vi "Build.vi"(4 "Build Specification Version":T1, 6 "Destination":path=path "Module Plugin Distribution", 7 "String in":refnum<vi>, 8 "error in":errorcluster, 9 "BuildSpecification":path=path "Module Plugin Distribution", 10 "Project":path=path "C:/temp/Workspace/Components/Modules/Data Collector Report Models/External/JSON/DC - JSON.lvproj", 11 "WorkspaceFolder":path=path "C:/temp/Workspace") -> (0 "error out":errorcluster)   [LabVIEW 2017]
uses:
  <vilib>/AppBuilder/AB_API_Simple/Build Specification Version.ctl
  <vilib>/AppBuilder/AB_API_Simple/Set Build Specification Version (path).vi
  <vilib>/AppBuilder/AB_API_Simple/Build (path).vi
  <vilib>/AppBuilder/AB_API/SDIST/NI_AB_API_SDIST.lvclass
  <vilib>/AppBuilder/AB_API/PPL/NI_AB_API_PPL.lvclass
  <vilib>/AppBuilder/AB_API_Simple/NI_App_Builder_API.lvlib
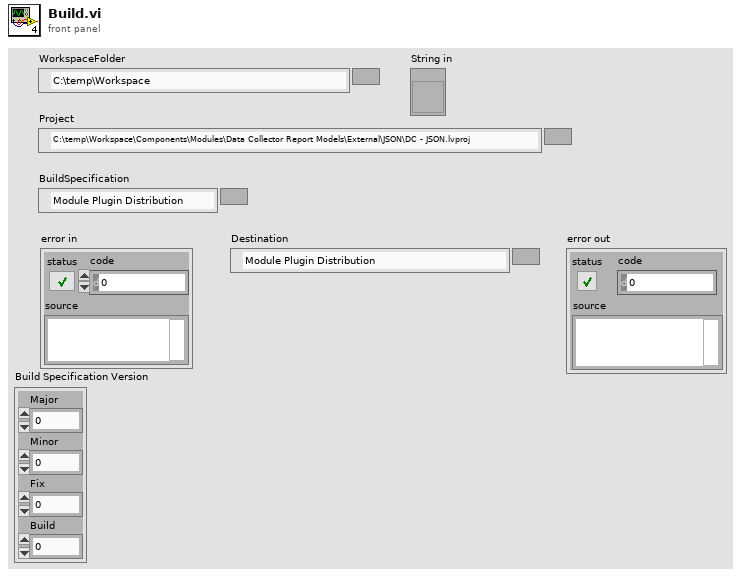
[diagram p1: front panel]
types:
  T1 = typedef "NI_App_Builder_API.lvlib/Build Specification Version.ctl" = cluster{"Major":u16, "Minor":u16, "Fix":u16, "Build":u16}
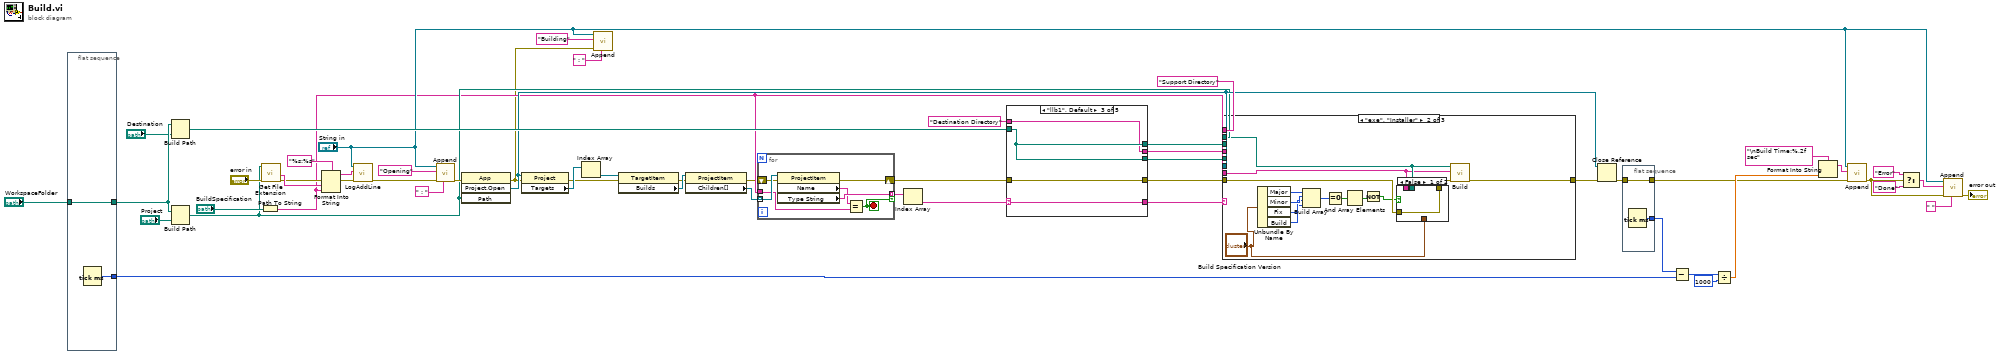
[diagram p0: block diagram]
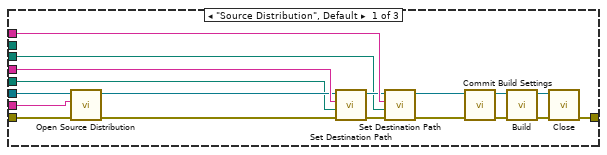
[diagram p2: hidden frame]
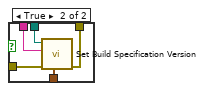
[diagram p3: hidden frame]
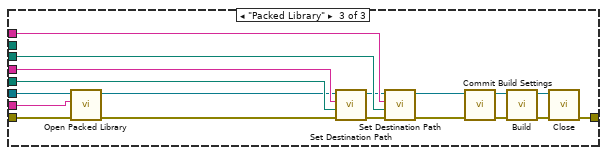
[diagram p4: hidden frame]
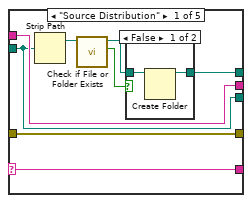
[diagram p5: hidden frame]
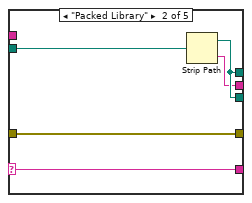
[diagram p7: hidden frame]
diagram:
  n1 = flat-sequence {
    tunnel: [w58] -> w25
    tunnel: "WorkspaceFolder" -> [w58]
    tunnel: [w57] -> w20
    frame #0 {
      n2 = Tick Count (ms)() -> (millisecond timer value=w57:u32)
    }
  }
  n3 = Build Path(base path=w25, name or relative path="Destination") -> (appended path=w47:path)
  n4 = Build Path(base path=w25, name or relative path="Project") -> (appended path=w12:path)
  n5 = Path To String(path="BuildSpecification") -> (string=w9:string)
  n6 = call <vilib>:"Get File Extension.vi"("error in (no error)"="error in", "file"=w12) -> ("error out"=w45:errorcluster, "filename without extension"=w50:string)  [unwired: 5 in, 3 out]
  n7 = Format Into String(format string="%s:%s", error in=w45, w50, w9) -> (resulting string=w28:string, error out=w30:errorcluster)  [unwired: 1 in]
  n8 = call "LogAddLine.vi"("error in (no error)"=w30, "Msg in"=w28, "String in"="String in") -> ("error out"=w29:errorcluster)  [unwired: 6 in, 1 out]
  n9 = call "Append.vi"("separator"=" : ", "error in (no error)"=w29, "Msg in"="Opening" ("format string"), "String in"="String in") -> ("error out"=w35:errorcluster)  [unwired: 6 in]
  n10 = invoke class="App" method="Project.Open"(error in=w35, "Path"=w12) -> (error out=w5:errorcluster, "Project:Open"=w39:refnum<vi>)  [unwired: 2 in, 2 out]
  n11 = property class="Project"(reference=w39, error in=w5) -> (error out=w4:errorcluster, "Targets"=w38:refnum<vi>[])  [unwired: 1 out]
  n12 = Index Array(array=w38) -> (element=w37:refnum<vi>)  [unwired: 1 in]
  n13 = call "Append.vi"("separator"=" : ", "error in (no error)"=w5, "Msg in"="Building" ("format string"), "String in"="String in") -> ()  [unwired: 6 in, 1 out]
  n14 = property class="TargetItem"(reference=w37, error in=w4) -> (error out=w3:errorcluster, "Builds"=w36:refnum<vi>)  [unwired: 1 out]
  n15 = property class="ProjectItem"(reference=w36, error in=w3) -> (error out=w2:errorcluster, "Children[]"=w10:refnum<vi>[])  [unwired: 1 out]
  n16 = for {
    tunnel: [w65] -> w8 mode=indexing if=w61
    tunnel: w10 -> [w64] mode=indexing
    tunnel: w9 -> [w62]
    shift-right: [w59] -> w1
    shift-left: w2 -> [w60]
    stop <- w61 stop-if-true
    n17 = property class="ProjectItem"(reference=w64, error in=w60) -> (error out=w59:errorcluster, "Name"=w63:string, "Type String"=w65:string)  [unwired: 1 out]
    n18 = Equal?(x=w63, y=w62) -> (x = y?=w61:bool)
  }
  n19 = Index Array(array=w8) -> (element=w7:string)  [unwired: 1 in]
  n20 = case shown="\"llb1\", Default" w7 {
    selector: w7 -> [w67 w78 w83 w87 w91]
    tunnel: [w72 w80 w85 w89 w92] -> w46
    tunnel: w47 -> [w72 w81 w85 w89 w92]
    tunnel: [w68 w80 w85 w89 w92] -> w44
    tunnel: [w67 w78 w83 w87 w91] -> w43
    tunnel: [w73 w79 w84 w88 w93] -> w41
    tunnel: "Destination Directory" ("Destination label") -> [w73 _ w84 w88 w93]
    tunnel: [w66 w77 w82 w86 w90] -> w6
    tunnel: w1 -> [w66 w77 w82 w86 w90]
    frame "Source Distribution" {
      n21 = Strip Path(path=w72) -> (stripped path=w69:path)  [unwired: 1 out]
      n22 = call <vilib>:"Check if File or Folder Exists.vi"("path"=w69) -> ("file or folder exists?"=w71:bool, "dup path"=w70:path)  [unwired: 8 in, 1 out]
      n23 = case shown="False" w71 {
        tunnel: w70 -> [w75 w76]
        tunnel: [w74 w76] -> w68
        frame False {
          n24 = Create Folder(path (use dialog)=w75) -> (created path=w74:path)  [unwired: 2 in, 2 out]
        }
        frame True {
        }
      }
    }
    frame "Packed Library" {
      n25 = Strip Path(path=w81) -> (stripped path=w80:path, name=w79:string)
    }
    frame "llb1", Default {
    }
    frame "exe" {
    }
    frame "" {
    }
  }
  n26 = case shown="\"exe\", \"Installer\"" w43 {
    tunnel: [w107 w125 w140] -> w42
    tunnel: w41 -> [w106 _ w148]
    tunnel: "Support Directory" ("Destination label") -> [w103 _ w146]
    tunnel: w46 -> [w98 _ w149]
    tunnel: w44 -> [w97 _ w145]
    tunnel: w6 -> [w96 w122 w139]
    tunnel: w39 -> [w95 _ w138]
    tunnel: w9 -> [w94 w123 w137]
    tunnel: w12 -> [_ w124 _]
    frame "Source Distribution", Default {
      n27 = call <vilib>:"Open Source Distribution.vi"("error in (no error)"=w96, "Build specification name"=w94, "Project Refnum"=w95) -> ("error out"=w104:errorcluster, "SDIST out"=w105:refnum<class "NI_AB_API_SDIST.lvclass">)  [unwired: 7 in]
      n28 = call-dynamic "Set Destination Path.vi"("error in (no error)"=w104, "Destination path"=w98, "Destination label"=w106, "SDIST in"=w105) -> ("error out"=w101:errorcluster, "SDIST out"=w102:refnum<class "NI_AB_API_SDIST.lvclass">)  [unwired: 6 in]
      n29 = call-dynamic "Set Destination Path.vi"("error in (no error)"=w101, "Destination path"=w97, "Destination label"=w103, "SDIST in"=w102) -> ("error out"=w100:errorcluster, "SDIST out"=w99:refnum<class "NI_AB_API_SDIST.lvclass">)  [unwired: 6 in]
      n30 = call-dynamic "Commit Build Settings.vi"("error in (no error)"=w100, "SDIST in"=w99) -> ("error out"=w111:errorcluster, "SDIST out"=w110:refnum<class "NI_AB_API_SDIST.lvclass">)  [unwired: 8 in]
      n31 = call-dynamic <vilib>:"Build.vi"("error in (no error)"=w111, "SDIST in"=w110) -> ("error out"=w109:errorcluster, "SDIST out"=w108:refnum<class "NI_AB_API_SDIST.lvclass">)  [unwired: 6 in, 2 out]
      n32 = call-dynamic "Close.vi"("error in (no error)"=w109, "SDIST in"=w108) -> ("error out"=w107:errorcluster)  [unwired: 9 in]
    }
    frame "exe", "Installer" {
      n33 = Unbundle By Name("Build Specification Version") -> ("Major"=w120:u16, "Minor"=w119:u16, "Fix"=w117:u16, "Build"=w118:u16)
      n34 = Build Array(w120, w119, w118, w117) -> (w116:u16[])
      n35 = Equal To 0?(x=w116) -> (x = 0?=w115:bool[])
      n36 = And Array Elements(Boolean array=w115) -> (logical AND=w114:bool)
      n37 = Not(x=w114) -> (.not. x?=w113:bool)
      n38 = case shown="False" w113 {
        tunnel: w124 -> [_ w131]
        tunnel: w123 -> [_ w130]
        tunnel: w122 -> [w126 w129]
        tunnel: [w126 w128] -> w121
        tunnel: "Build Specification Version" -> [_ w127]
        frame False {
        }
        frame True {
          n39 = call-poly <vilib>:"Set Build Specification Version.vi"("Build Specification Version"=w127, "error in (no error)"=w129, "Name of build specification"=w130, "Path to project"=w131) -> ("error out"=w128:errorcluster)  [unwired: 7 in]
        }
      }
      n40 = call-poly <vilib>:"Build.vi"("error in (no error)"=w121, "Name of build specification (if empty: build all)"=w123, "Path to project"=w124) -> ("error out"=w125:errorcluster)  [unwired: 7 in, 1 out]
    }
    frame "Packed Library" {
      n41 = call <vilib>:"Open Packed Library.vi"("error in (no error)"=w139, "Build specification name"=w137, "Project Refnum"=w138) -> ("error out"=w135:errorcluster, "PPL out"=w136:refnum<class "NI_AB_API_PPL.lvclass">)  [unwired: 7 in]
      n42 = call-dynamic "Set Destination Path.vi"("error in (no error)"=w135, "Destination path"=w149, "Destination label"=w148, "PPL in"=w136) -> ("error out"=w147:errorcluster, "PPL out"=w134:refnum<class "NI_AB_API_PPL.lvclass">)  [unwired: 6 in]
      n43 = call-dynamic "Set Destination Path.vi"("error in (no error)"=w147, "Destination path"=w145, "Destination label"=w146, "PPL in"=w134) -> ("error out"=w133:errorcluster, "PPL out"=w132:refnum<class "NI_AB_API_PPL.lvclass">)  [unwired: 6 in]
      n44 = call-dynamic "Commit Build Settings.vi"("error in (no error)"=w133, "PPL in"=w132) -> ("error out"=w143:errorcluster, "PPL out"=w144:refnum<class "NI_AB_API_PPL.lvclass">)  [unwired: 8 in]
      n45 = call-dynamic <vilib>:"Build.vi"("error in (no error)"=w143, "PPL in"=w144) -> ("error out"=w141:errorcluster, "PPL out"=w142:refnum<class "NI_AB_API_PPL.lvclass">)  [unwired: 6 in, 2 out]
      n46 = call-dynamic "Close.vi"("error in (no error)"=w141, "DLL in"=w142) -> ("error out"=w140:errorcluster)  [unwired: 9 in]
    }
  }
  n47 = Close Reference(reference=w39, error in (no error)=w42) -> (error out=w24:errorcluster)
  n48 = flat-sequence {
    tunnel: [w151] -> w15
    tunnel: w24 -> [w151]
    tunnel: [w150] -> w21
    frame #0 {
      n49 = Tick Count (ms)() -> (millisecond timer value=w150:u32)
    }
  }
  n50 = Subtract(x=w21, y=w20) -> (x-y=w19:u32)
  n51 = Divide(x=w19, y=u32 1000) -> (x/y=w17:dbl)
  n52 = Format Into String(format string="\nBuild Time:%.2f sec", w17) -> (resulting string=w16:string)  [unwired: 2 in, 1 out]
  n53 = call "Append.vi"("error in (no error)"=w15, "Msg in"=w16, "String in"="String in") -> ("error out"=w14:errorcluster)  [unwired: 7 in]
  n54 = Select(t="Error" ("f"), s=w14, f="Done" ("Msg in")) -> (s? t:f=w54:string)
  n55 = call "Append.vi"("separator"=" ", "error in (no error)"=w14, "Msg in"=w54, "String in"="String in") -> ("error out"=→"error out":errorcluster)  [unwired: 6 in]
